vi "GEOM_GUI.vi"() -> ()   [LabVIEW 2016]
panel:
  in  "reload":bool
  in  "detnum":bool
  out "fpainfo":string
  in  "Defined Headers":i32(listbox)
  in  "Amplifiers Location":i32(listbox)
  out "yslide":u32(slide) scale=-1.0..4112.0
  out "xslide":u32(slide) scale=-1.0..4211.084337349397
  in  "get modif":bool
  in  "Modifiers":i32(listbox)
  in  "change value":i32
  in  "DETECTOR INFO":i32(listbox)
  in  "FPA INFO":i32(listbox)
  out "zoom":dbl
  in  "stop":bool
  in  "readmode":u16(ring) items=["lowerleft", "lowerright", "upperright", "upperleft", "lower", "upper", "quad"]
  in  "name":string(combo)
  out "FPA":picture
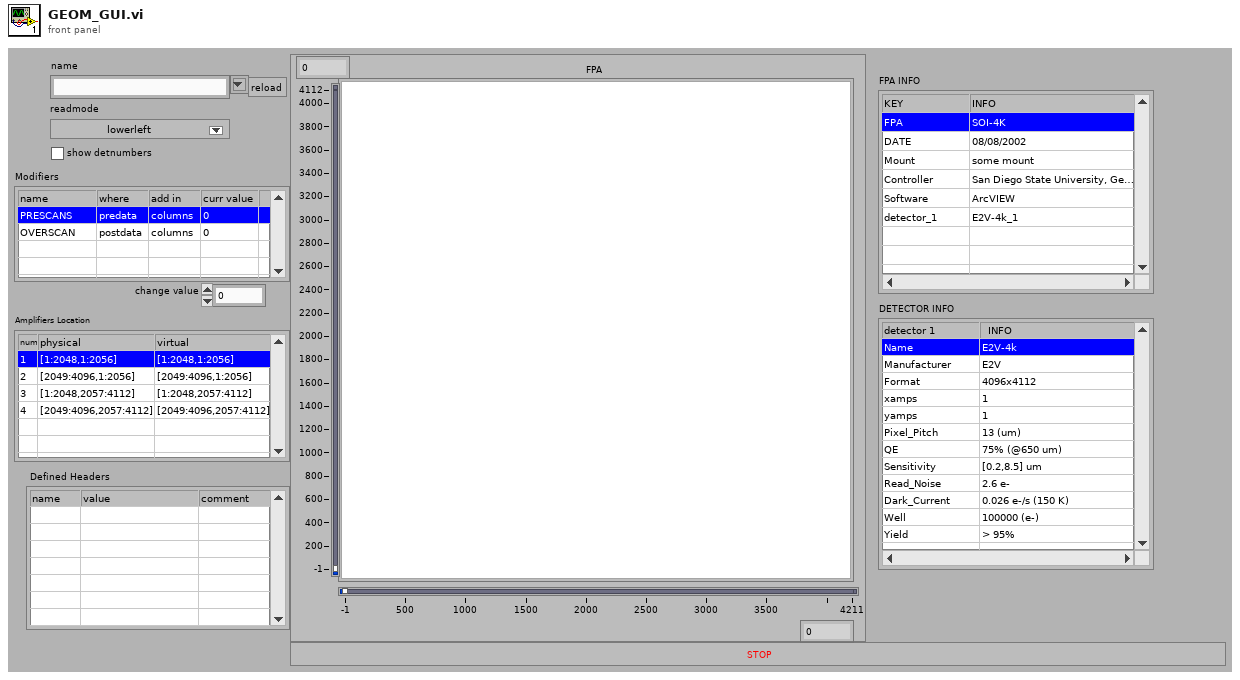
[diagram p1: front panel]
types:
  T1 = typedef "GEOM_AmpModifiers.ctl" = cluster{"Binning":T2, "sections":T3[]}
  T2 = typedef "GEOM_Binning.ctl" = cluster{"x":u32, "y":u32}
  T3 = typedef "GEOM_Moifier.ctl" = cluster{"name":string, "header section":string, "comment":string, "value":i32, "binning?":bool, "Where":enum16{"predata", "postdata"}, "add In":enum16{"columns", "rows", "none"}}
  T4 = typedef "LVBoundsTypeDef.ctl" = cluster{"Width":u32, "Height":u32}
  T5 = typedef "GEOM_CorrectedFPA.ctl" = cluster{"readmode":string, "amplifiers":cluster{"number":i32, "xstart":i32, "ystart":i32}[], "totxsize":i32, "totysize":i32, "maxxdim":i32, "maxydim":i32, "numxamps":i32, "numyamps":i32, "totxdata":i32, "totydata":i32, "xdataamp":i32, "ydataamp":i32, "totpixels":i32}
  T6 = typedef "GEOM_Amplifier.ctl" = cluster{"number":i32, "type":T7, "rotated":i16, "fliped":u16, "FPAcoord":cluster{"xstart":i32, "ystart":i32}, "Physical_size":cluster{"columns":i32, "rows":i32}, "predata":cluster{"columns":i32, "rows":i32}, "postdata":cluster{"columns":i32, "rows":i32}, "Req ROIs":T8, "Corr ROI":T8, "Detnumber":i32, "ampID":string, "discard":i32}
  T7 = typedef "GEOM_AmpType.ctl" = u16
  T8 = typedef "GEOM_ROI.ctl" = T9[]
  T9 = typedef "GEOM_Coords.ctl" = cluster{"xstart":u32, "ystart":u32, "xsize":u32, "ysize":u32}
  T10 = cluster{"number":i32, "xstart":i32, "ystart":i32}[]
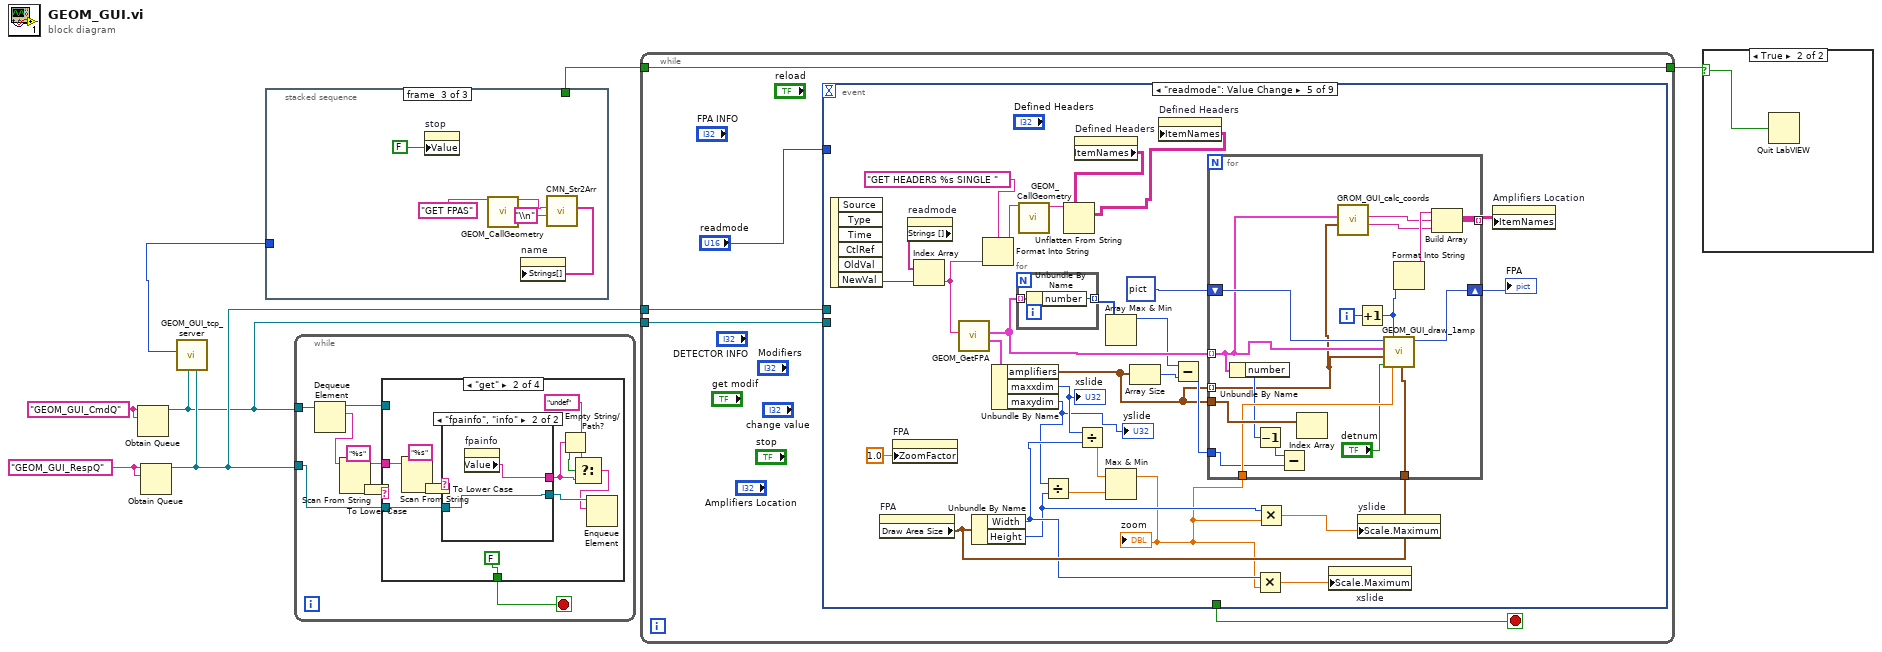
[diagram p0: block diagram]
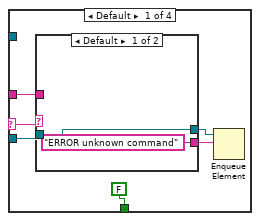
[diagram p2: hidden frame]
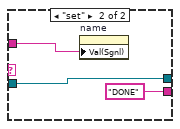
[diagram p3: hidden frame]
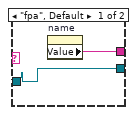
[diagram p4: hidden frame]
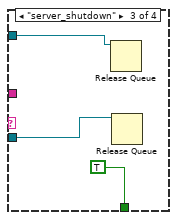
[diagram p5: hidden frame]
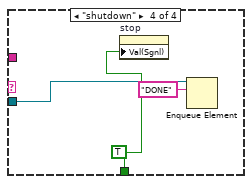
[diagram p6: hidden frame]
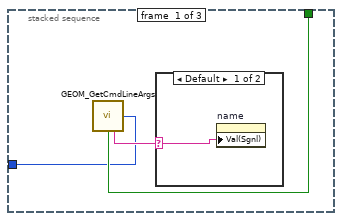
[diagram p8: hidden frame]
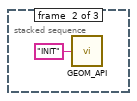
[diagram p10: hidden frame]
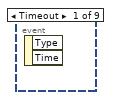
[diagram p11: hidden frame]
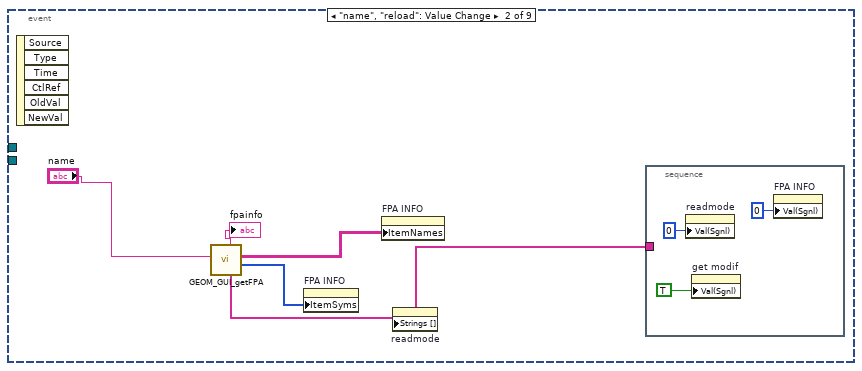
[diagram p12: hidden frame]
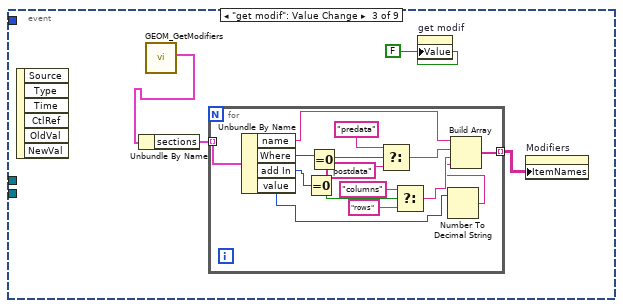
[diagram p13: hidden frame]
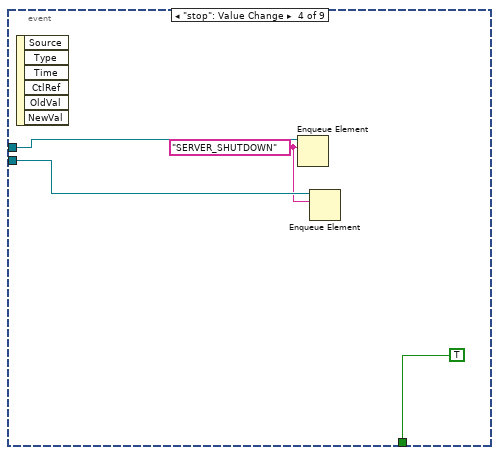
[diagram p14: hidden frame]
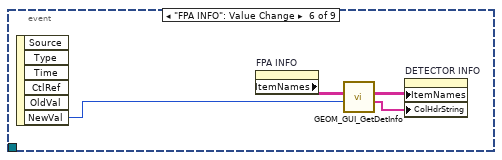
[diagram p15: hidden frame]
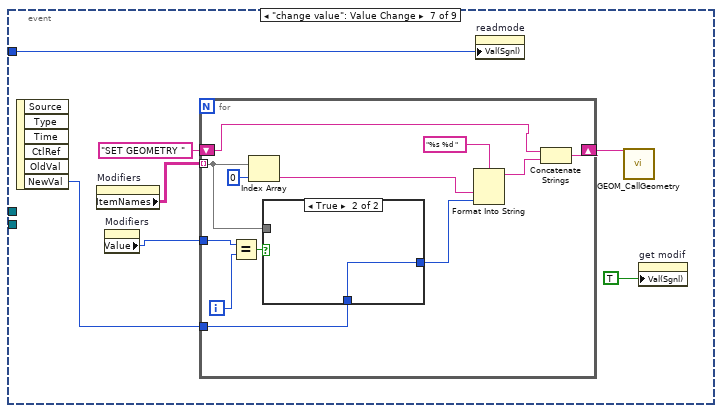
[diagram p16: hidden frame]
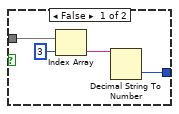
[diagram p17: hidden frame]
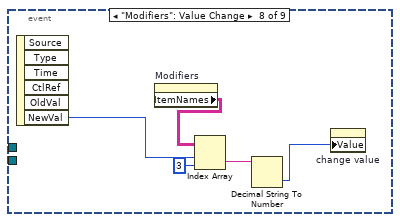
[diagram p18: hidden frame]
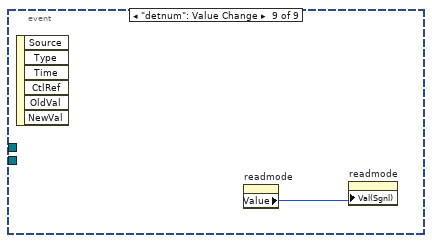
[diagram p19: hidden frame]
diagram:
  w4 = "GEOM_GUI_RespQ" ("name (unnamed)")
  w5 = "GEOM_GUI_CmdQ" ("name (unnamed)")
  n1 = Obtain Queue(name (unnamed)=w5, element data type=w5) -> (queue out=w2:refnum<queue>)  [unwired: 3 in, 2 out]
  n2 = Obtain Queue(name (unnamed)=w4, element data type=w4) -> (queue out=w3:refnum<queue>)  [unwired: 3 in, 2 out]
  n3 = stacked-sequence {
    tunnel: [w9 _ _] -> w7
    tunnel: [w8 _ _] -> w1
    frame #0 {
      n4 = call "GEOM_GetCmdLineArgs.vi"() -> ("port"=w8:u16, "exit"=w9:bool, "fpa"=w10:string)  [unwired: 13 out]
      n5 = case shown="Default" w10 {
        selector: w10 -> [w11 _]
        frame Default {
          n6 = property on="name" class="CmbBox"("Val(Sgnl)"=w11) -> ()  [unwired: 2 in, 2 out]
        }
        frame "_undef_" {
        }
      }
    }
    frame #1 {
      n7 = call "GEOM_API.vi"("Cmd"="INIT") -> ()  [unwired: 1 in, 14 out]
    }
    frame #2 {
      n8 = property on="stop" class="Bool (strict)"("Value"=FALSE ("stop")) -> ()  [unwired: 2 in, 2 out]
      n9 = call "GEOM_CallGeometry.vi"("Command"="GET FPAS" ("Cmd")) -> ("ImmedReplyString"=w16:string)  [unwired: 1 in, 13 out]
      n10 = call "CMN_Str2Arr.vi"("separator"="\\n", "string in"=w16) -> ("Array out"=w14:string[])  [unwired: 2 in, 7 out]
      n11 = property on="name" class="CmbBox"("Strings[]"=w14) -> ()  [unwired: 2 in, 2 out]
    }
  }
  n12 = call "GEOM_GUI_tcp_server.vi"("resp queue"=w3, "from sock queue"=w2, "port"=w1) -> ()  [unwired: 9 out]
  n13 = while {
    tunnel: w2 -> [w26]
    tunnel: w3 -> [w22]
    stop <- w23 stop-if-true
    n14 = Dequeue Element(queue=w26) -> (queue out=w21:refnum<queue>, element=w19:string)  [unwired: 1 in, 3 out]
    n15 = Scan From String(format string="%s", input string=w19) -> (remaining string=w20:string, output 1=w24:string)  [unwired: 2 in, 3 out]
    n16 = To Lower Case(string=w24) -> (all lower case string=w18:string)
    n17 = case shown="\"get\"" w18 {
      selector: w18 -> [w30 _ _ _]
      tunnel: [FALSE FALSE TRUE w58] -> w23
      tunnel: w22 -> [w31 w47 w54 w57]
      tunnel: w21 -> [_ _ w53 _]
      tunnel: w20 -> [w29 w45 _ _]
      frame Default {
        n18 = case shown="Default" w30 {
          tunnel: w31 -> [w34 w35]
          tunnel: w29 -> [_ w37]
          tunnel: ["ERROR unknown command" ("element") "DONE" ("element")] -> w28
          tunnel: [w34 w35] -> w27
          frame Default {
          }
          frame "set" {
            n19 = property on="name" class="CmbBox"("Val(Sgnl)"=w37) -> ()  [unwired: 2 in, 2 out]
          }
        }
        n20 = Enqueue Element(queue=w27, element=w28) -> ()  [unwired: 1 in, 4 out]
      }
      frame "get" {
        n21 = Scan From String(format string="%s", input string=w45) -> (output 1=w44:string)  [unwired: 2 in, 4 out]
        n22 = To Lower Case(string=w44) -> (all lower case string=w38:string)
        n23 = case shown="\"fpainfo\", \"info\"" w38 {
          tunnel: w47 -> [w50 w52]
          tunnel: [w50 w52] -> w43
          tunnel: [w49 w51] -> w42
          frame "fpa", Default {
            n24 = property on="name" class="CmbBox"() -> ("Value"=w49:string)  [unwired: 2 in, 2 out]
          }
          frame "fpainfo", "info" {
            n25 = property on="fpainfo" class="Str"() -> ("Value"=w51:string)  [unwired: 2 in, 2 out]
          }
        }
        n26 = Empty String/Path?(string/path=w42) -> (empty?=w40:bool)
        n27 = Select(t="undef", s=w40, f=w42) -> (s? t:f=w41:string)
        n28 = Enqueue Element(queue=w43, element=w41) -> ()  [unwired: 1 in, 4 out]
      }
      frame "server_shutdown" {
        n29 = Release Queue(queue=w53) -> ()  [unwired: 1 in, 4 out]
        n30 = Release Queue(queue=w54) -> ()  [unwired: 1 in, 4 out]
      }
      frame "shutdown" {
        w58 = TRUE
        n31 = property on="stop" class="Bool (strict)"("Val(Sgnl)"=w58) -> ()  [unwired: 2 in, 2 out]
        n32 = Enqueue Element(queue=w57, element="DONE") -> ()  [unwired: 1 in, 4 out]
      }
    }
  }
  n33 = while {
    tunnel: w7 -> [w61]
    tunnel: [w61] -> w6
    tunnel: w3 -> [w60]
    tunnel: w2 -> [w59]
    stop <- w63 stop-if-true
    n34 = event shown="[4] \"readmode\": Value Change" {
      selector: _ -> [_ _ _ _ _ _ _ _ _]
      dyn-events: _ -> [_ _ _ _ _ _ _ _ _]
      timeout: _ -> [_ _ _ _ _ _ _ _ _]
      tunnel: [_ _ _ TRUE _ _ _ _ _] -> w63
      tunnel: "readmode" -> [_ _ _ _ _ _ w149 _ _]
      tunnel: w60 -> [_ _ _ w93 _ _ _ _ _]
      tunnel: w59 -> [_ _ _ w92 _ _ _ _ _]
      event Timeout {
        n35 = event-data() -> ()  [unwired: 3 out]
      }
      event "name", "reload": Value Change {
        n36 = event-data() -> ()  [unwired: 7 out]
        n37 = call "GEOM_GUI_getFPA.vi"("name"="name") -> ("items"=w67:i32[], "fpa info"=w66:string[][], "readmodes"=w65:string[], "fpainfo"=→"fpainfo":string)  [unwired: 7 out]
        n38 = property on="FPA INFO" class="MCListbox (strict)"("ItemSyms"=w67) -> ()  [unwired: 2 in, 2 out]
        n39 = property on="FPA INFO" class="MCListbox (strict)"("ItemNames"=w66) -> ()  [unwired: 2 in, 2 out]
        n40 = property on="readmode" class="Ring (strict)"("Strings []"=w65) -> ()  [unwired: 2 in, 2 out]
        n41 = stacked-sequence {
          tunnel: w65 -> [_]
          frame #0 {
            n42 = property on="readmode" class="Ring (strict)"("Val(Sgnl)"=u16 0 ("Value (Signaling)")) -> ()  [unwired: 2 in, 2 out]
            n43 = property on="get modif" class="Bool (strict)"("Val(Sgnl)"=TRUE ("Value (Signaling)")) -> ()  [unwired: 2 in, 2 out]
            n44 = property on="FPA INFO" class="MCListbox (strict)"("Val(Sgnl)"=0 ("Value (Signaling)")) -> ()  [unwired: 2 in, 2 out]
          }
        }
      }
      event "get modif": Value Change {
        n45 = event-data() -> ()  [unwired: 7 out]
        n46 = call "GEOM_GetModifiers.vi"() -> ("GEOM_modifiers"=w75:T1)  [unwired: 1 in, 10 out]
        n47 = Unbundle By Name(w75) -> ("sections"=w74:T3[])
        n48 = for {
          tunnel: w74 -> [w90] mode=indexing
          tunnel: [w76] -> w73 mode=indexing
          n49 = Unbundle By Name(w90) -> ("name"=w81:string, "Where"=w89:enum16{"predata", "postdata"}, "add In"=w87:enum16{"columns", "rows", "none"}, "value"=w77:i32)
          n50 = Equal To 0?(x=w87) -> (x = 0?=w86:bool)
          n51 = Equal To 0?(x=w89) -> (x = 0?=w88:bool)
          n52 = Select(t="predata", s=w88, f="postdata") -> (s? t:f=w80:string)
          n53 = Select(t="columns", s=w86, f="rows") -> (s? t:f=w79:string)
          n54 = Number To Decimal String(number=w77) -> (decimal integer string=w78:string)  [unwired: 1 out]
          n55 = Build Array(w81, w80, w79, w78) -> (w76:string[])
        }
        n56 = property on="get modif" class="Bool (strict)"("Value"=FALSE ("get modif")) -> ()  [unwired: 2 in, 2 out]
        n57 = property on="Modifiers" class="MCListbox (strict)"("ItemNames"=w73) -> ()  [unwired: 2 in, 2 out]
      }
      event "stop": Value Change {
        w91 = "SERVER_SHUTDOWN" ("element")
        n58 = event-data() -> ()  [unwired: 7 out]
        n59 = Enqueue Element(queue=w93, element=w91) -> ()  [unwired: 1 in, 4 out]
        n60 = Enqueue Element(queue=w92, element=w91) -> ()  [unwired: 1 in, 4 out]
      }
      event "readmode": Value Change {
        n61 = event-data() -> ("NewVal"=w122:u16)  [unwired: 6 out]
        n62 = property on="FPA" class="Pict"() -> ("Draw Area Size"=w116:T4)  [unwired: 2 in, 2 out]
        n63 = property on="FPA" class="Pict"("ZoomFactor"=sgl 1.0 ("Zoom Factor")) -> ()  [unwired: 2 in, 2 out]
        n64 = property on="readmode" class="Ring (strict)"() -> ("Strings []"=w123:string[])  [unwired: 2 in, 2 out]
        n65 = Index Array(array=w123, index=w122) -> (element=w102:string)
        n66 = call "GEOM_GetFPA.vi"("readmode"=w102) -> ("CorrectedFPACoord"=w121:T5, "amplifiers"=w99:T6[])  [unwired: 2 in, 7 out]
        n67 = Unbundle By Name(w116) -> ("Width"=w114:u32, "Height"=w110:u32)
        n68 = Format Into String(format string="GET HEADERS %s SINGLE " ("Command"), w102) -> (resulting string=w101:string)  [unwired: 2 in, 1 out]
        n69 = Unbundle By Name(w121) -> ("amplifiers"=w95:T10, "maxxdim"=w112:i32, "maxydim"=w111:i32)
        "xslide" <- w112
        "yslide" <- w111
        n70 = for {
          tunnel: w99 -> [w125] mode=indexing
          tunnel: [w124] -> w100 mode=indexing
          n71 = Unbundle By Name(w125) -> ("number"=w124:i32)
        }
        n72 = call "GEOM_CallGeometry.vi"("Command"=w101) -> ("ImmedReplyString"=w106:string)  [unwired: 1 in, 13 out]
        n73 = Divide(x=w111, y=w110) -> (x/y=w119:dbl)
        n74 = property on="Defined Headers" class="MCListbox (strict)"() -> ("ItemNames"=w105:string[][])  [unwired: 2 in, 2 out]
        n75 = Unflatten From String(type=w105, binary string=w106) -> (value=w104:string[][])  [unwired: 1 in, 4 out]
        n76 = Divide(x=w112, y=w114) -> (x/y=w120:dbl)
        n77 = Array Max & Min(array=w100) -> (max value=w98:i32)  [unwired: 3 out]
        n78 = Max & Min(x=w120, y=w119) -> (max(x,y)=w109:dbl)  [unwired: 1 out]
        "zoom" <- w109
        n79 = Array Size(array=w95) -> (size(s)=w97:i32)
        n80 = property on="Defined Headers" class="MCListbox (strict)"("ItemNames"=w104) -> ()  [unwired: 2 in, 2 out]
        n81 = Subtract(x=w98, y=w97) -> (x-y=w96:i32)
        n82 = for {
          tunnel: w99 -> [w137] mode=indexing
          shift-right: [w141] -> w117
          shift-left: picture data[5B] ("new picture") -> [w142]
          tunnel: w116 -> [w140]
          tunnel: w109 -> [w132]
          tunnel: w95 -> [w139]
          tunnel: [w133] -> w107 mode=indexing
          tunnel: w96 -> [w130]
          tunnel: w95 -> [w127] mode=indexing
          i -> [w138]
          n83 = Unbundle By Name(w137) -> ("number"=w129:i32)
          n84 = Decrement(x=w129) -> (x-1=w131:i32)
          n85 = Subtract(x=w131, y=w130) -> ()  [unwired: 1 out]
          n86 = Index Array(array=w139) -> ()  [unwired: 1 in, 1 out]
          n87 = call "GROM_GUI_calc_coords.vi"("corr amps"=w127, "amps"=w137) -> ("virt coords"=w134:string, "phys coords"=w135:string)  [unwired: 8 out]
          n88 = Increment(x=w138) -> (x+1=w128:i32)
          n89 = call "GEOM_GUI_draw_1amp.vi"("zoom factor"=w132, "picture size"=w140, "order"=w128, "detnum"="detnum", "corr amps"=w127, "amps"=w137, "picture in"=w142) -> ("picture out"=w141:picture)  [unwired: 1 in, 3 out]
          n90 = Format Into String(w128) -> (resulting string=w136:string)  [unwired: 3 in, 1 out]
          n91 = Build Array(w136, w135, w134) -> (w133:string[])
        }
        "FPA" <- w117
        n92 = Multiply(x=w114, y=w109) -> (x*y=w113:dbl)
        n93 = Multiply(x=w110, y=w109) -> (x*y=w108:dbl)
        n94 = property on="xslide" class="Slide (strict)"("Scale.Maximum"=w113) -> ()  [unwired: 2 in, 2 out]
        n95 = property on="yslide" class="Slide (strict)"("Scale.Maximum"=w108) -> ()  [unwired: 2 in, 2 out]
        n96 = property on="Amplifiers Location" class="MCListbox (strict)"("ItemNames"=w107) -> ()  [unwired: 2 in, 2 out]
      }
      event "FPA INFO": Value Change {
        n97 = event-data() -> ("NewVal"=w145:i32)  [unwired: 6 out]
        n98 = property on="FPA INFO" class="MCListbox (strict)"() -> ("ItemNames"=w146:string[][])  [unwired: 2 in, 2 out]
        n99 = call "GEOM_GUI_GetDetInfo.vi"("index"=w145, "fpa info in"=w146) -> ("col headers"=w143:string[], "item names"=w144:string[][])  [unwired: 8 out]
        n100 = property on="DETECTOR INFO" class="MCListbox (strict)"("ItemNames"=w144, "ColHdrString"=w143) -> ()  [unwired: 2 in, 2 out]
      }
      event "change value": Value Change {
        n101 = event-data() -> ("NewVal"=w151:i32)  [unwired: 6 out]
        n102 = property on="Modifiers" class="MCListbox (strict)"() -> ("ItemNames"=w153:string[][])  [unwired: 2 in, 2 out]
        n103 = property on="Modifiers" class="MCListbox (strict)"() -> ("Value"=w147:i32)  [unwired: 2 in, 2 out]
        n104 = for {
          tunnel: w153 -> [w161] mode=indexing
          tunnel: w147 -> [w164]
          shift-right: [w156] -> w150
          shift-left: "SET GEOMETRY " -> [w155]
          tunnel: w151 -> [w154]
          i -> [w163]
          n105 = Equal?(x=w164, y=w163) -> (x = y?=w162:bool)
          n106 = Index Array(array=w161, index=0) -> (element=w158:string)
          n107 = case shown="True" w162 {
            tunnel: w161 -> [w169 _]
            tunnel: [w166 w170] -> w159
            tunnel: w154 -> [_ w170]
            frame False {
              n108 = Index Array(array=w169, index=3) -> (element=w167:string)
              n109 = Decimal String To Number(string=w167) -> (number=w166:i32)  [unwired: 3 out]
            }
            frame True {
            }
          }
          n110 = Format Into String(format string="%s %d ", w158, w159) -> (resulting string=w157:string)  [unwired: 2 in, 1 out]
          n111 = Concatenate Strings(w155, w157) -> (w156:string)
        }
        n112 = property on="readmode" class="Ring (strict)"("Val(Sgnl)"=w149) -> ()  [unwired: 2 in, 2 out]
        n113 = call "GEOM_CallGeometry.vi"("Command"=w150) -> ()  [unwired: 1 in, 14 out]
        n114 = property on="get modif" class="Bool (strict)"("Val(Sgnl)"=TRUE ("Value (Signaling)")) -> ()  [unwired: 2 in, 2 out]
      }
      event "Modifiers": Value Change {
        n115 = event-data() -> ("NewVal"=w174:i32)  [unwired: 6 out]
        n116 = property on="Modifiers" class="MCListbox (strict)"() -> ("ItemNames"=w175:string[][])  [unwired: 2 in, 2 out]
        n117 = Index Array(array=w175, index (row)=w174, index (col)=3 ("disabled index (col)")) -> (element=w172:string)
        n118 = Decimal String To Number(string=w172) -> (number=w171:i32)  [unwired: 3 out]
        n119 = property on="change value" class="DigNum (strict)"("Value"=w171) -> ()  [unwired: 2 in, 2 out]
      }
      event "detnum": Value Change {
        n120 = event-data() -> ()  [unwired: 7 out]
        n121 = property on="readmode" class="Ring (strict)"() -> ("Value"=w176:u16)  [unwired: 2 in, 2 out]
        n122 = property on="readmode" class="Ring (strict)"("Val(Sgnl)"=w176) -> ()  [unwired: 2 in, 2 out]
      }
    }
  }
  n123 = case shown="True" w6 {
    selector: w6 -> [_ w177]
    frame False {
    }
    frame True {
      n124 = Quit LabVIEW(quit? (T)=w177) -> ()
    }
  }
